vi "Msg.vi"(7 "Actor in":refnum<class "Actor.lvclass">, 11 "Teardown Msg in":refnum<class "Teardown Msg.lvclass">) -> (5 "Actor out":refnum<class "Actor.lvclass">)   [LabVIEW 2021, in "jettl.lvlib" / "Teardown.lvlib" / "Teardown Msg.lvclass"]
uses:
  Teardown Msg.lvclass
  jettl/Actor/Actor.lvclass
  Teardown/Teardown.lvclass
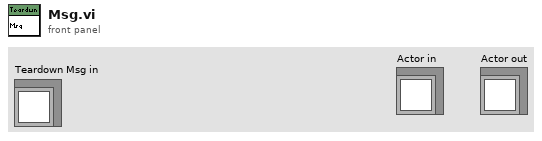
[diagram p1: front panel]
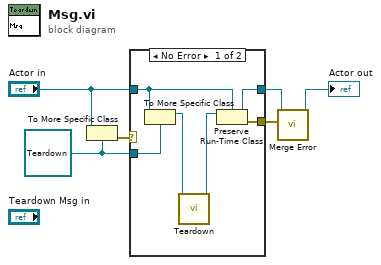
[diagram p0: block diagram]
diagram:
  w3 = refnum<class "Teardown.lvclass"> refnum ("Destroy.lvlib:Destroy.lvclass")
  n1 = To More Specific Class(target class=w3, reference="Actor in") -> (error out=w6:errorcluster)  [unwired: 1 in, 1 out]
  n2 = case shown="No Error" w6 {
    selector: w6 -> [_ w13]
    tunnel: [w10 w14] -> w4
    tunnel: "Actor in" -> [w11 w14]
    tunnel: w3 -> [w12 _]
    tunnel: [w9 w13] -> w5
    frame No Error {
      n3 = To More Specific Class(target class=w12, reference=w11) -> (specific class reference=w8:refnum<class "Teardown.lvclass">)  [unwired: 1 in, 1 out]
      n4 = call-dynamic "Teardown.vi"("Teardown in"=w8) -> ("Teardown out"=w7:refnum<class "Teardown.lvclass">)  [unwired: 10 in]
      n5 = Preserve Run-Time Class(object in=w7, 2:w11) -> (object out=w10:refnum<class "Actor.lvclass">, error out=w9:errorcluster)  [unwired: 1 in]
    }
    frame Error {
    }
  }
  n6 = call-dynamic "Merge Error.vi"("Error"=w5, "Set Error in"=w4) -> ("Set Error out"=→"Actor out":refnum<class "Actor.lvclass">)  [unwired: 9 in]
